vi "Set Units METRIC.vi"(8 "error in":errorcluster, 11 "Vaisala in":refnum<class "Vaisala.lvclass">) -> (0 "error out":errorcluster, 3 "Vaisala out":refnum<class "Vaisala.lvclass">)   [LabVIEW 2014, in "Vaisala.lvclass"]
uses:
  Vaisala.lvclass
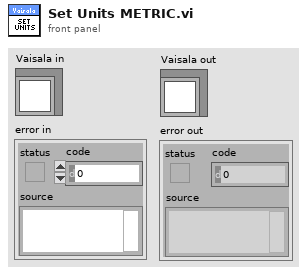
[diagram p1: front panel]
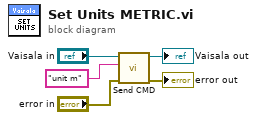
[diagram p0: block diagram]
diagram:
  n1 = call-dynamic "Send CMD.vi"("error in"="error in", "CMD In"="unit m" ("Write - Async"), "Vaisala in"="Vaisala in") -> ("error out"=→"error out":errorcluster, "Vaisala out"=→"Vaisala out":refnum<class "Vaisala.lvclass">)  [unwired: 7 in]
